vi "Remove File Extension.vi"(7 "filename":string) -> (2 "extension":string, 3 "adjustedfilename":string)   [LabVIEW 2009, in "File IO.lvclass"]
uses:
  File IO.lvclass
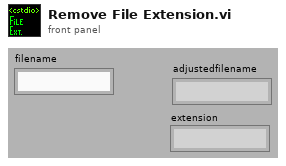
[diagram p1: front panel]
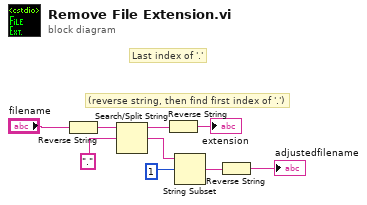
[diagram p0: block diagram]
diagram:
  # "(reverse string, then find first index of '.')"
  # "Last index of '.'"
  n1 = Reverse String(1:"filename") -> (0:w5:string)
  n2 = Search/Split String(string=w5, search string/char (-)=".") -> (substring before match=w4:string, match + rest of string=w8:string)  [unwired: 2 out]
  n3 = Reverse String(1:w4) -> (0:→"extension":string)
  n4 = String Subset(string=w8, offset (0)=1) -> (substring=w2:string)  [unwired: 1 out]
  n5 = Reverse String(1:w2) -> (0:→"adjustedfilename":string)
